vi "Determine More Warnings.vi"() -> ()   [LabVIEW 2014]
panel:
  in  "Max Wind Speed":dbl
  in  "Current Wind Speed":dbl
  out "Warning Text":string
  out "Boolean":bool
  in  "Current Temp":dbl
  in  "Min Temp":dbl
  in  "Max Temp":dbl
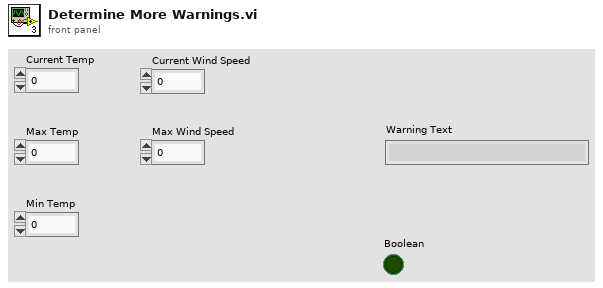
[diagram p1: front panel]
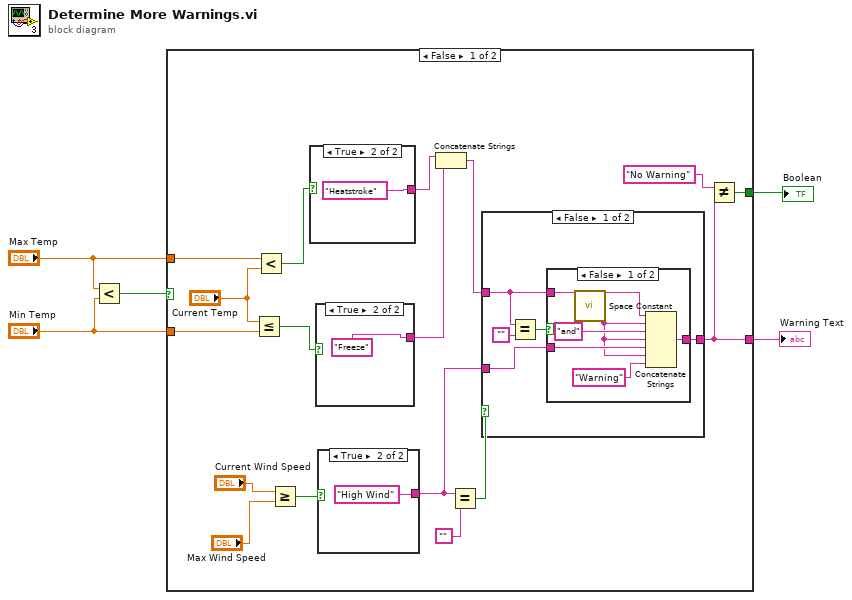
[diagram p0: block diagram]
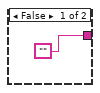
[diagram p2: hidden frame]
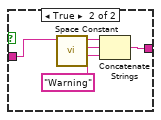
[diagram p3: hidden frame]
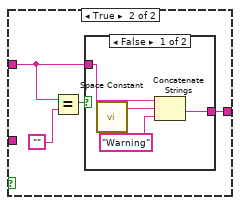
[diagram p4: hidden frame]
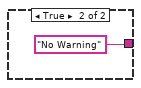
[diagram p5: hidden frame]
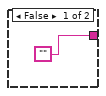
[diagram p6: hidden frame]
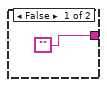
[diagram p7: hidden frame]
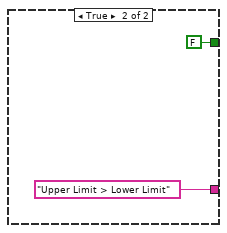
[diagram p8: hidden frame]
diagram:
  n1 = Less?(x="Max Temp", y="Min Temp") -> (x < y?=w5:bool)
  n2 = case shown="False" w5 {
    tunnel: "Min Temp" -> [w17 _]
    tunnel: "Max Temp" -> [w16 _]
    tunnel: [w8 "Upper Limit > Lower Limit"] -> w2
    tunnel: [w7 FALSE] -> w1
    frame False {
      n3 = Less Or Equal?(x="Current Temp", y=w17) -> (x <= y?=w22:bool)
      n4 = Less?(x=w16, y="Current Temp") -> (x < y?=w21:bool)
      n5 = Greater Or Equal?(x="Current Wind Speed", y="Max Wind Speed") -> (x >= y?=w12:bool)
      n6 = case shown="True" w21 {
        tunnel: ["" "Heatstroke"] -> w19
        frame False {
        }
        frame True {
        }
      }
      n7 = case shown="True" w22 {
        tunnel: ["" "Freeze"] -> w18
        frame False {
        }
        frame True {
        }
      }
      n8 = case shown="True" w12 {
        tunnel: ["" "High Wind"] -> w6
        frame False {
        }
        frame True {
        }
      }
      n9 = Concatenate Strings(w19, w18) -> (w20:string)
      n10 = Equal?(x=w6, y="") -> (x = y?=w13:bool)
      n11 = case shown="False" w13 {
        tunnel: w20 -> [w27 w40]
        tunnel: [w29 w42] -> w8
        tunnel: w6 -> [w25 _]
        frame False {
          n12 = Equal?(x=w27, y="") -> (x = y?=w28:bool)
          n13 = case shown="False" w28 {
            tunnel: [w35 w39] -> w29
            tunnel: w27 -> [w34 _]
            tunnel: w25 -> [w31 w38]
            frame False {
              n14 = call <vilib>:"Space Constant.vi"() -> ("String"=w30:string)
              n15 = Concatenate Strings(w34, w30, "and", w30, w31, w30, "Warning") -> (w35:string)
            }
            frame True {
              n16 = call <vilib>:"Space Constant.vi"() -> ("String"=w37:string)
              n17 = Concatenate Strings(w38, w37, "Warning" ("string")) -> (w39:string)
            }
          }
        }
        frame True {
          n18 = Equal?(x=w40, y="") -> (x = y?=w43:bool)
          n19 = case shown="False" w43 {
            tunnel: [w47 "No Warning"] -> w42
            tunnel: w40 -> [w46 _]
            frame False {
              n20 = call <vilib>:"Space Constant.vi"() -> ("String"=w45:string)
              n21 = Concatenate Strings(w46, w45, "Warning" ("string")) -> (w47:string)
            }
            frame True {
            }
          }
        }
      }
      n22 = Not Equal?(x="No Warning", y=w8) -> (x != y?=w7:bool)
    }
    frame True {
    }
  }
  "Boolean" <- w1
  "Warning Text" <- w2
